vi "Add Elements.vi"(7 "Element 2":string, 11 "Element 1":string) -> (3 "Sum":string)   [LabVIEW 2021]
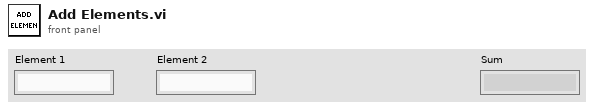
[diagram p1: front panel]
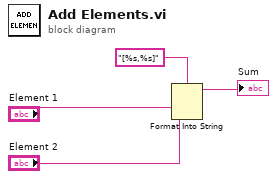
[diagram p0: block diagram]
diagram:
  n1 = Format Into String(format string="[%s,%s]", "Element 1", "Element 2") -> (resulting string=→"Sum":string)  [unwired: 2 in, 1 out]
